vi "Get List of PINs - TOI.vi"(11 "Test Configuration":T2={"Target Pout Per Tone (dBm)"=0.0, "Start Value"={"Power Level per Tone (dBm)"=0.0, "Center Frequency (Hz)"=0.0, "Tone Spacing (Hz)"=0.0}, "Sweep Settings"={"Mode"=enum."Power", "Sweep Delay (ms)"=0, "Power Sweep End"=-20.0, "Power Sweep Step"=-20.0, "Frequency Sweep End"=-4.0, "Frequency Sweep Step"=1.0, "Tone Spacing Sweep End"=-4.0, "Tone Spacing Sweep Step"=1.0}} {"Sweep Settings"."Tone Spacing Sweep Step" format="%#.pHz"; "Sweep Settings"."Tone Spacing Sweep End" format="%#.pHz"; "Sweep Settings"."Frequency Sweep Step" format="%#.pHz"; "Sweep Settings"."Frequency Sweep End" format="%#.pHz"; "Sweep Settings"."Power Sweep End" format="%#_6p"; "Sweep Settings"."Sweep Delay (ms)" format="%#.3p"; "Start Value"."Tone Spacing (Hz)" format="%#_6p"; "Start Value"."Center Frequency (Hz)" format="%#.3p"}) -> (2 "Sweep List":T1[](array[typedef]), 3 "Test Configuration out":T2={"Target Pout Per Tone (dBm)"=0.0, "Start Value"={"Power Level per Tone (dBm)"=0.0, "Center Frequency (Hz)"=0.0, "Tone Spacing (Hz)"=0.0}, "Sweep Settings"={"Mode"=enum."Power", "Sweep Delay (ms)"=0, "Power Sweep End"=-20.0, "Power Sweep Step"=-20.0, "Frequency Sweep End"=-4.0, "Frequency Sweep Step"=1.0, "Tone Spacing Sweep End"=-4.0, "Tone Spacing Sweep Step"=1.0}} {"Sweep Settings"."Tone Spacing Sweep Step" format="%#.pHz"; "Sweep Settings"."Tone Spacing Sweep End" format="%#.pHz"; "Sweep Settings"."Frequency Sweep Step" format="%#.pHz"; "Sweep Settings"."Frequency Sweep End" format="%#.pHz"; "Sweep Settings"."Power Sweep End" format="%#_6p"; "Sweep Settings"."Sweep Delay (ms)" format="%#.3p"; "Start Value"."Tone Spacing (Hz)" format="%#_6p"; "Start Value"."Center Frequency (Hz)" format="%#.3p"})   [LabVIEW 2023]
uses:
  Controls/Test Config - TOI.ctl
  Controls/Data Cluster - Settings - TOI.ctl
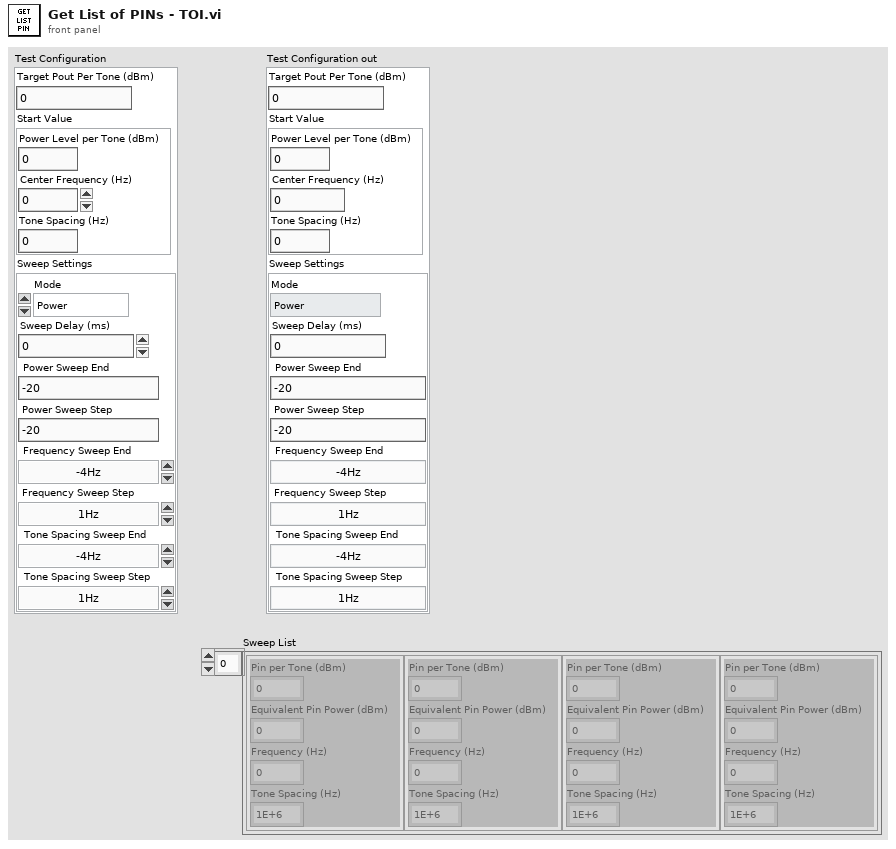
[diagram p1: front panel]
types:
  T1 = typedef "Data Cluster - Settings - TOI.ctl" = cluster{"Pin per Tone (dBm)":dbl, "Equivalent Pin Power (dBm)":dbl, "Frequency (Hz)":dbl, "Tone Spacing (Hz)":dbl}
  T2 = typedef "Test Config - TOI.ctl" = cluster{"Target Pout Per Tone (dBm)":dbl, "Start Value":cluster{"Power Level per Tone (dBm)":dbl, "Center Frequency (Hz)":dbl, "Tone Spacing (Hz)":dbl}, "Sweep Settings":cluster{"Mode":enum16{"Power", "Frequency", "Tone Spacing"}, "Sweep Delay (ms)":u32, "Power Sweep End":dbl, "Power Sweep Step":dbl, "Frequency Sweep End":dbl, "Frequency Sweep Step":dbl, "Tone Spacing Sweep End":dbl, "Tone Spacing Sweep Step":dbl}}
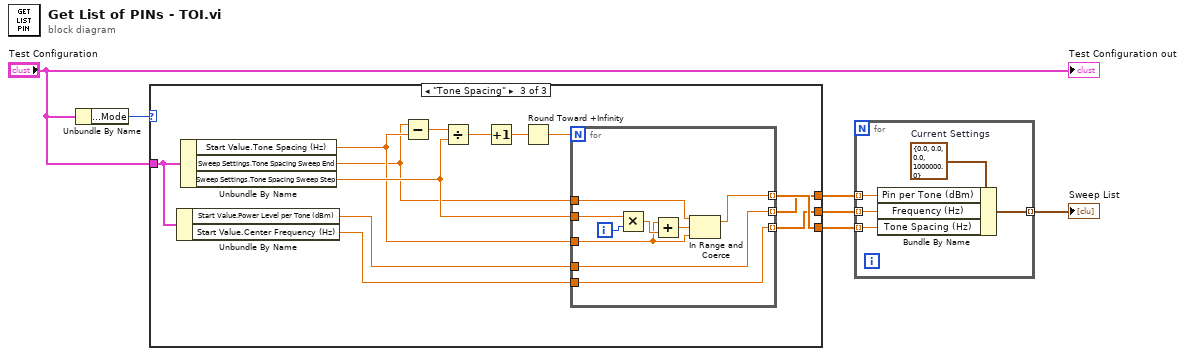
[diagram p0: block diagram]
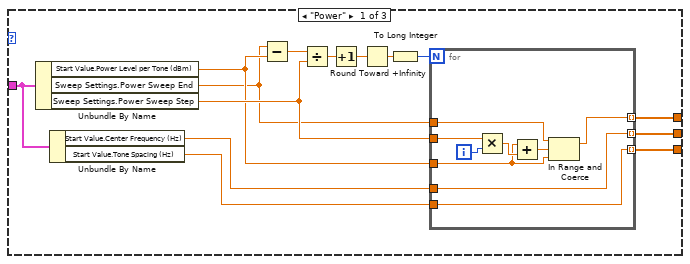
[diagram p2: hidden frame]
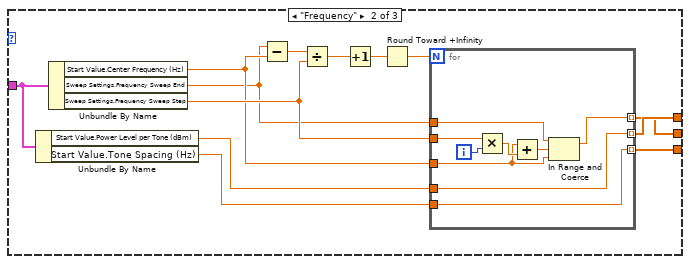
[diagram p3: hidden frame]
diagram:
  n1 = Unbundle By Name("Test Configuration") -> ("Sweep Settings.Mode"=w5:enum16{"Power", "Frequency", "Tone Spacing"})
  n2 = case shown="\"Tone Spacing\"" w5 {
    tunnel: "Test Configuration" -> [w20 w42 w64]
    tunnel: [w10 w31 w53] -> w4
    tunnel: [w9 w30 w52] -> w3
    tunnel: [w8 w32 w54] -> w2
    frame "Power" {
      n3 = Unbundle By Name(w20) -> ("Start Value.Power Level per Tone (dBm)"=w18:dbl, "Sweep Settings.Power Sweep End"=w17:dbl, "Sweep Settings.Power Sweep Step"=w19:dbl)
      n4 = Unbundle By Name(w20) -> ("Start Value.Center Frequency (Hz)"=w12:dbl, "Start Value.Tone Spacing (Hz)"=w11:dbl)
      n5 = Subtract(x=w17, y=w18) -> (x-y=w14:dbl)
      n6 = Divide(x=w14, y=w19) -> (x/y=w13:dbl)
      n7 = Increment(x=w13) -> (x+1=w15:dbl)
      n8 = Round Toward +Infinity(x=w15) -> (ceil(x): smallest int >= x=w16:dbl)
      n9 = To Long Integer(number=w16) -> (32bit integer=w7:i32)
      n10 = for {
        N: w7 -> [_]
        tunnel: w17 -> [w25]
        tunnel: w19 -> [w27]
        tunnel: w18 -> [w24]
        tunnel: w12 -> [w22]
        tunnel: w11 -> [w21]
        tunnel: [w23] -> w10 mode=indexing
        tunnel: [w22] -> w9 mode=indexing
        tunnel: [w21] -> w8 mode=indexing
        i -> [w28]
        n11 = Multiply(x=w27, y=w28) -> (x*y=w29:dbl)
        n12 = Add(x=w24, y=w29) -> (x+y=w26:dbl)
        n13 = In Range and Coerce(upper limit=w25, x=w26, lower limit=w24) -> (coerced(x)=w23:dbl)  [unwired: 1 out]
      }
    }
    frame "Frequency" {
      n14 = Unbundle By Name(w42) -> ("Start Value.Power Level per Tone (dBm)"=w34:dbl, "Start Value.Tone Spacing (Hz)"=w33:dbl)
      n15 = Unbundle By Name(w42) -> ("Start Value.Center Frequency (Hz)"=w40:dbl, "Sweep Settings.Frequency Sweep End"=w39:dbl, "Sweep Settings.Frequency Sweep Step"=w41:dbl)
      n16 = Subtract(x=w39, y=w40) -> (x-y=w36:dbl)
      n17 = Divide(x=w36, y=w41) -> (x/y=w35:dbl)
      n18 = Increment(x=w35) -> (x+1=w37:dbl)
      n19 = Round Toward +Infinity(x=w37) -> (ceil(x): smallest int >= x=w38:dbl)
      n20 = for {
        N: w38 -> [_]
        tunnel: w39 -> [w47]
        tunnel: w41 -> [w49]
        tunnel: w40 -> [w46]
        tunnel: w34 -> [w44]
        tunnel: w33 -> [w43]
        tunnel: [w45] -> w30 mode=indexing
        tunnel: [w44] -> w31 mode=indexing
        tunnel: [w43] -> w32 mode=indexing
        i -> [w50]
        n21 = Multiply(x=w49, y=w50) -> (x*y=w51:dbl)
        n22 = Add(x=w46, y=w51) -> (x+y=w48:dbl)
        n23 = In Range and Coerce(upper limit=w47, x=w48, lower limit=w46) -> (coerced(x)=w45:dbl)  [unwired: 1 out]
      }
    }
    frame "Tone Spacing" {
      n24 = Unbundle By Name(w64) -> ("Start Value.Power Level per Tone (dBm)"=w56:dbl, "Start Value.Center Frequency (Hz)"=w55:dbl)
      n25 = Unbundle By Name(w64) -> ("Start Value.Tone Spacing (Hz)"=w62:dbl, "Sweep Settings.Tone Spacing Sweep End"=w61:dbl, "Sweep Settings.Tone Spacing Sweep Step"=w63:dbl)
      n26 = Subtract(x=w61, y=w62) -> (x-y=w58:dbl)
      n27 = Divide(x=w58, y=w63) -> (x/y=w57:dbl)
      n28 = Increment(x=w57) -> (x+1=w59:dbl)
      n29 = Round Toward +Infinity(x=w59) -> (ceil(x): smallest int >= x=w60:dbl)
      n30 = for {
        N: w60 -> [_]
        tunnel: w61 -> [w69]
        tunnel: w63 -> [w71]
        tunnel: w62 -> [w68]
        tunnel: w56 -> [w66]
        tunnel: w55 -> [w65]
        tunnel: [w67] -> w54 mode=indexing
        tunnel: [w66] -> w53 mode=indexing
        tunnel: [w65] -> w52 mode=indexing
        i -> [w72]
        n31 = Multiply(x=w71, y=w72) -> (x*y=w73:dbl)
        n32 = Add(x=w68, y=w73) -> (x+y=w70:dbl)
        n33 = In Range and Coerce(upper limit=w69, x=w70, lower limit=w68) -> (coerced(x)=w67:dbl)  [unwired: 1 out]
      }
    }
  }
  n34 = for {
    tunnel: w4 -> [w77] mode=indexing
    tunnel: w3 -> [w76] mode=indexing
    tunnel: w2 -> [w75] mode=indexing
    tunnel: [w74] -> w1 mode=indexing
    w78 = T1 {"Pin per Tone (dBm)"=0.0, "Equivalent Pin Power (dBm)"=0.0, "Frequency (Hz)"=0.0, "Tone Spacing (Hz)"=1000000.0}  # Current Settings
    n35 = Bundle By Name(cluster=w78, "Pin per Tone (dBm)"=w77, "Frequency (Hz)"=w76, "Tone Spacing (Hz)"=w75) -> (w74:T1)
  }
  "Sweep List" <- w1
  "Test Configuration out" <- "Test Configuration"
